vi "ReleaseQueue.vi"(8 "error in (no error)":errorcluster, 11 "PriorityQueue in":refnum<class "PriorityQueue.lvclass">) -> (0 "error out":errorcluster)   [LabVIEW 2019, in "PriorityQueue.lvclass"]
doc: "Releases the PriorityQueue resources."
uses:
  PriorityQueue.lvclass
  PriorityQueue.lvclass/PriorityQueue.ctl
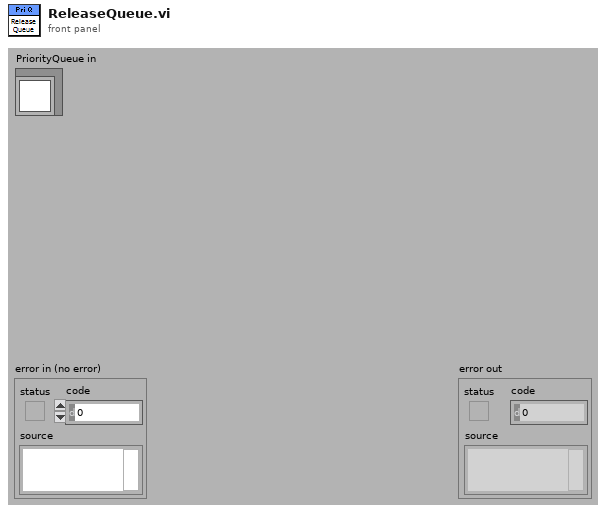
[diagram p1: front panel]
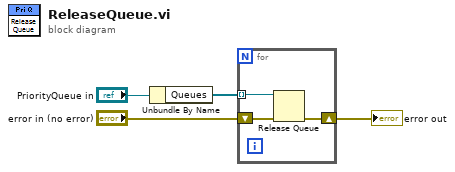
[diagram p0: block diagram]
diagram:
  n1 = Unbundle By Name("PriorityQueue in") -> ("Queues"=w3:refnum<queue>[])
  n2 = for {
    tunnel: w3 -> [w7] mode=indexing
    shift-right: [w5] -> w1
    shift-left: "error in (no error)" -> [w6]
    n3 = Release Queue(queue=w7, error in (no error)=w6) -> (error out=w5:errorcluster)  [unwired: 1 in, 2 out]
  }
  "error out" <- w1
